vi "update_position.vi"(8 "error in (no error)":errorcluster, 11 "FH090410SharedVariableStage in":refnum<class "StageFH090410SharedVariable.lvclass">) -> (0 "error out":errorcluster, 3 "FH090410SharedVariableStage out":refnum<class "StageFH090410SharedVariable.lvclass">)   [LabVIEW 2010, in "StageFH090410SharedVariable.lvclass"]
uses:
  StageFH090410SharedVariable.lvclass
  StageFH090410SharedVariable.lvclass/StageFH090410SharedVariable.ctl
  StageDL090409Scaffold/StageDL090409Scaffold/StageDL090409Scaffold.lvclass
  common/classes/SpaceVector/SpaceVector/SpaceVector.lvclass
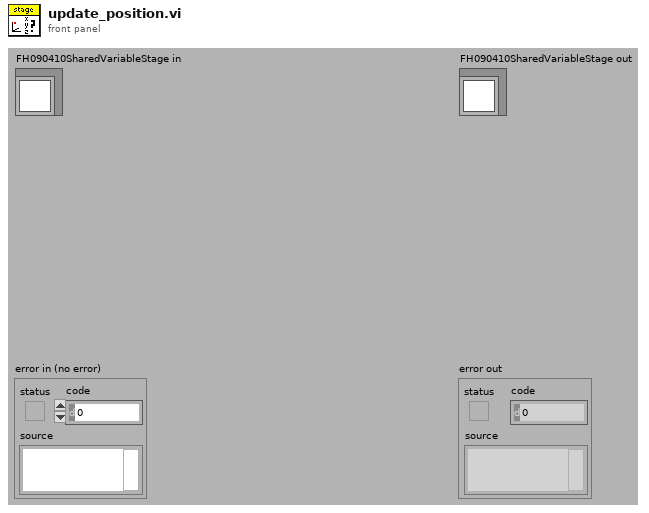
[diagram p1: front panel]
types:
  T1 = typedef "space_vector_cluster.ctl" = cluster{"x":dbl[unit], "y":dbl[unit], "z":dbl[unit]}
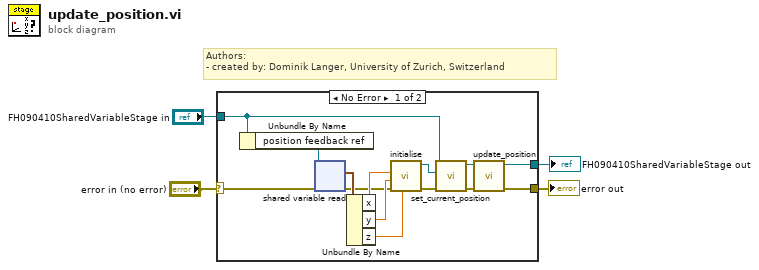
[diagram p0: block diagram]
diagram:
  # "Authors: \n- created by: Dominik Langer, University of Zurich, Switzerland"
  n1 = case shown="No Error" "error in (no error)" {
    selector: "error in (no error)" -> [w6 w20]
    tunnel: [w17 w20] -> w3
    tunnel: [w18 w19] -> w1
    tunnel: "FH090410SharedVariableStage in" -> [w16 w19]
    frame No Error {
      n2 = Unbundle By Name(w16) -> ("position feedback ref"=w7:refnum<k21>)
      n3 = shared-variable-read(w7, w6) -> (w5:errorcluster, w11:T1)  [unwired: 2 out]
      n4 = Unbundle By Name(w11) -> ("x"=w10:dbl[unit], "y"=w9:dbl[unit], "z"=w8:dbl[unit])
      n5 = call "initialise.vi"("z"=w8, "error in (no error)"=w5, "y"=w9, "x"=w10) -> ("error out"=w13:errorcluster, "SpaceVector out"=w12:refnum<class "SpaceVector.lvclass">)  [unwired: 6 out]
      n6 = call-dynamic "set_current_position.vi"("error in (no error)"=w13, "current position"=w12, "DL090409StageScaffold.lvclass in"=w16) -> ("error out"=w14:errorcluster, "DL090409StageScaffold.lvclass out"=w15:refnum<class "StageFH090410SharedVariable.lvclass">)  [unwired: 7 out]
      n7 = call-parent "update_position.vi"("error in (no error)"=w14, "DL090409StageScaffold in"=w15) -> ("error out"=w17:errorcluster, "DL090409StageScaffold out"=w18:refnum<class "StageFH090410SharedVariable.lvclass">)  [unwired: 8 out]
    }
    frame Error {
    }
  }
  "error out" <- w3
  "FH090410SharedVariableStage out" <- w1
